vi "Vision Server Get Timestamp.vi"() -> (0 "Timestamp (ms)":dbl)   [LabVIEW 2016]
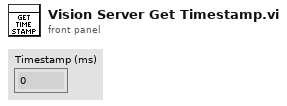
[diagram p1: front panel]
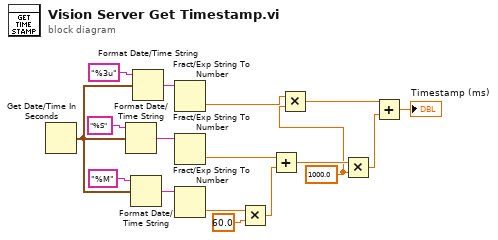
[diagram p0: block diagram]
diagram:
  w2 = 1000.0 ("y")
  n1 = Get Date/Time In Seconds() -> (seconds since 1Jan1904=w11:timestamp)
  n2 = Format Date/Time String(time format string (%c)="%S", seconds (now)=w11) -> (date/time string=w14:string)  [unwired: 1 in]
  n3 = Format Date/Time String(time format string (%c)="%M", seconds (now)=w11) -> (date/time string=w9:string)  [unwired: 1 in]
  n4 = Format Date/Time String(time format string (%c)="%3u", seconds (now)=w11) -> (date/time string=w15:string)  [unwired: 1 in]
  n5 = Fract/Exp String To Number(string=w15) -> (number=w3:dbl)  [unwired: 3 in, 1 out]
  n6 = Fract/Exp String To Number(string=w14) -> (number=w6:dbl)  [unwired: 3 in, 1 out]
  n7 = Fract/Exp String To Number(string=w9) -> (number=w8:dbl)  [unwired: 3 in, 1 out]
  n8 = Multiply(x=w8, y=60.0) -> (x*y=w5:dbl)
  n9 = Add(x=w6, y=w5) -> (x+y=w4:dbl)
  n10 = Multiply(x=w3, y=w2) -> (x*y=w1:dbl)
  n11 = Multiply(x=w4, y=w2) -> (x*y=w13:dbl)
  n12 = Add(x=w1, y=w13) -> (x+y=→"Timestamp (ms)":dbl)
